vi "Module (Top Level).vi"(8 "error in":errorcluster) -> (0 "error out":errorcluster)   [LabVIEW 2017, in "Game.lvlib"]
uses:
  Game.lvlib
  User Events/TypeDefs/Shutdown UE FGV Command.ctl
  Global TypeDefs/Registered Modules.ctl
  Public TypeDefs/Messages.ctl
  Public TypeDefs/Module Events.ctl
  Libraries/TypeDefs/WorkspaceConfig.ctl
  Libraries/TypeDefs/UserInfo.ctl
  Libraries/TypeDefs/ServerStreamData.ctl
  Libraries/TypeDefs/HandPosition.ctl
  Libraries/TypeDefs/ElbowPosition.ctl
  Libraries/TypeDefs/ShoulderPosition.ctl
  Libraries/TypeDefs/UserInput.ctl
  Public TypeDefs/Target Position.ctl
  Logger/Logger.lvlib
  Error Handler/Error Handler.lvlib
  Controller/Controller.lvlib
  Libraries/GameComms.lvlib
  mypam/myPAM.lvlib
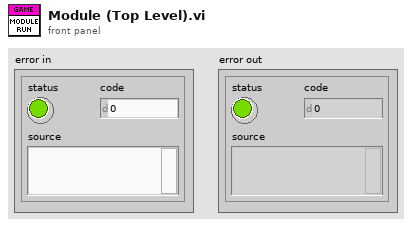
[diagram p1: front panel]
types:
  T1 = typedef "Registered Modules.ctl" = enum16{"Controller", "DAQ", "Error Handler", "Game", "myPAM", "WinHost", "Logger"}
  T2 = typedef "Shutdown UE FGV Command.ctl" = enum16{"create", "get", "destroy"}
  T3 = typedef "Controller.lvlib/Module Reference.ctl" = cluster{"calling module":T1, "module queues":T4, "module notifiers":T5}
  T4 = typedef "Controller.lvlib/Module Queues.ctl" = cluster{"message queue":refnum<queue>}
  T5 = typedef "Controller.lvlib/Module Notifiers.ctl" = cluster{"dummy notifier":refnum<notifier>}
  T6 = typedef "myPAM.lvlib/Module Reference.ctl" = cluster{"calling module":T1, "module queues":T7, "module notifiers":T8}
  T7 = typedef "myPAM.lvlib/Module Queues.ctl" = cluster{"message queue":refnum<queue>}
  T8 = typedef "myPAM.lvlib/Module Notifiers.ctl" = cluster{"end eff. pos.":refnum<notifier>}
  T9 = typedef "Logger.lvlib/Module Reference.ctl" = cluster{"calling module":T1, "module queues":T10, "module notifiers":T11}
  T10 = typedef "Logger.lvlib/Module Queues.ctl" = cluster{"message queue":refnum<queue>}
  T11 = typedef "Logger.lvlib/Module Notifiers.ctl" = cluster{"dummy notifier":refnum<notifier>}
  T12 = typedef "Game.lvlib/Module Reference.ctl" = cluster{"calling module":T1, "module queues":T13, "module notifiers":T14}
  T13 = typedef "Game.lvlib/Module Queues.ctl" = cluster{"message queue":refnum<queue>}
  T14 = typedef "Game.lvlib/Module Notifiers.ctl" = cluster{"dummy notifier":refnum<notifier>}
  T15 = typedef "Error Handler.lvlib/Module Reference.ctl" = cluster{"calling module":T1, "module queues":T16, "module notifiers":T17}
  T16 = typedef "Error Handler.lvlib/Module Queues.ctl" = cluster{"message queue":refnum<queue>}
  T17 = typedef "Error Handler.lvlib/Module Notifiers.ctl" = cluster{"dummy notifier":refnum<notifier>}
  T18 = typedef "Game.lvlib/Module Events.ctl" = enum16{"client connected", "client status change", "client disconnected"}
  T19 = typedef "Game.lvlib/GameComms.lvlib/ServerStreamData.ctl" = cluster{"hPos":T20, "ePos":T21, "sPos":T22, "uInput":T23}
  T20 = typedef "Game.lvlib/GameComms.lvlib/HandPosition.ctl" = cluster{"x":dbl, "y":dbl, "z":dbl}
  T21 = typedef "Game.lvlib/GameComms.lvlib/ElbowPosition.ctl" = cluster{"x":dbl, "y":dbl, "z":dbl}
  T22 = typedef "Game.lvlib/GameComms.lvlib/ShoulderPosition.ctl" = cluster{"x":dbl, "y":dbl, "z":dbl}
  T23 = typedef "Game.lvlib/GameComms.lvlib/UserInput.ctl" = cluster{"g":dbl}
  T24 = typedef "Game.lvlib/Target Position.ctl" = cluster{"x (mm)":dbl, "y (mm)":dbl}
  T25 = typedef "Game.lvlib/Messages.ctl" = enum16{"wait for client", "communicate", "shutdown"}
  T26 = typedef "Game.lvlib/GameComms.lvlib/UserInfo.ctl" = cluster{"id":string, "disabilityLevel ":dbl, "upperArmLength":dbl, "lowerArmLength":dbl}
  T27 = typedef "Game.lvlib/GameComms.lvlib/WorkspaceConfig.ctl" = cluster{"x":dbl, "y":dbl, "z":dbl}
  T28 = typedef "Game.lvlib/GameComms.lvlib/Connection.ctl" = cluster{"UDP Connection ID":refnum<k16>, "TCP Connection ID":refnum<k5>, "Remote UDP Port":u16, "Remote IP":u32}
  T29 = typedef "Game.lvlib/GameComms.lvlib/ClientStreamData.ctl" = cluster{"tPos":T30, "tWeight":dbl, "f":T31, "v":dbl}
  T30 = typedef "Game.lvlib/GameComms.lvlib/TargetPosition.ctl" = cluster{"x":dbl, "y":dbl, "z":dbl}
  T31 = typedef "Game.lvlib/GameComms.lvlib/ForceVector.ctl" = cluster{"x":dbl, "y":dbl, "z":dbl}
  T32 = typedef "Game.lvlib/GameComms.lvlib/ClientStatusData.ctl" = cluster{"gameState":u16, "playerName":string, "playerScore":dbl, "gameUnits":string}
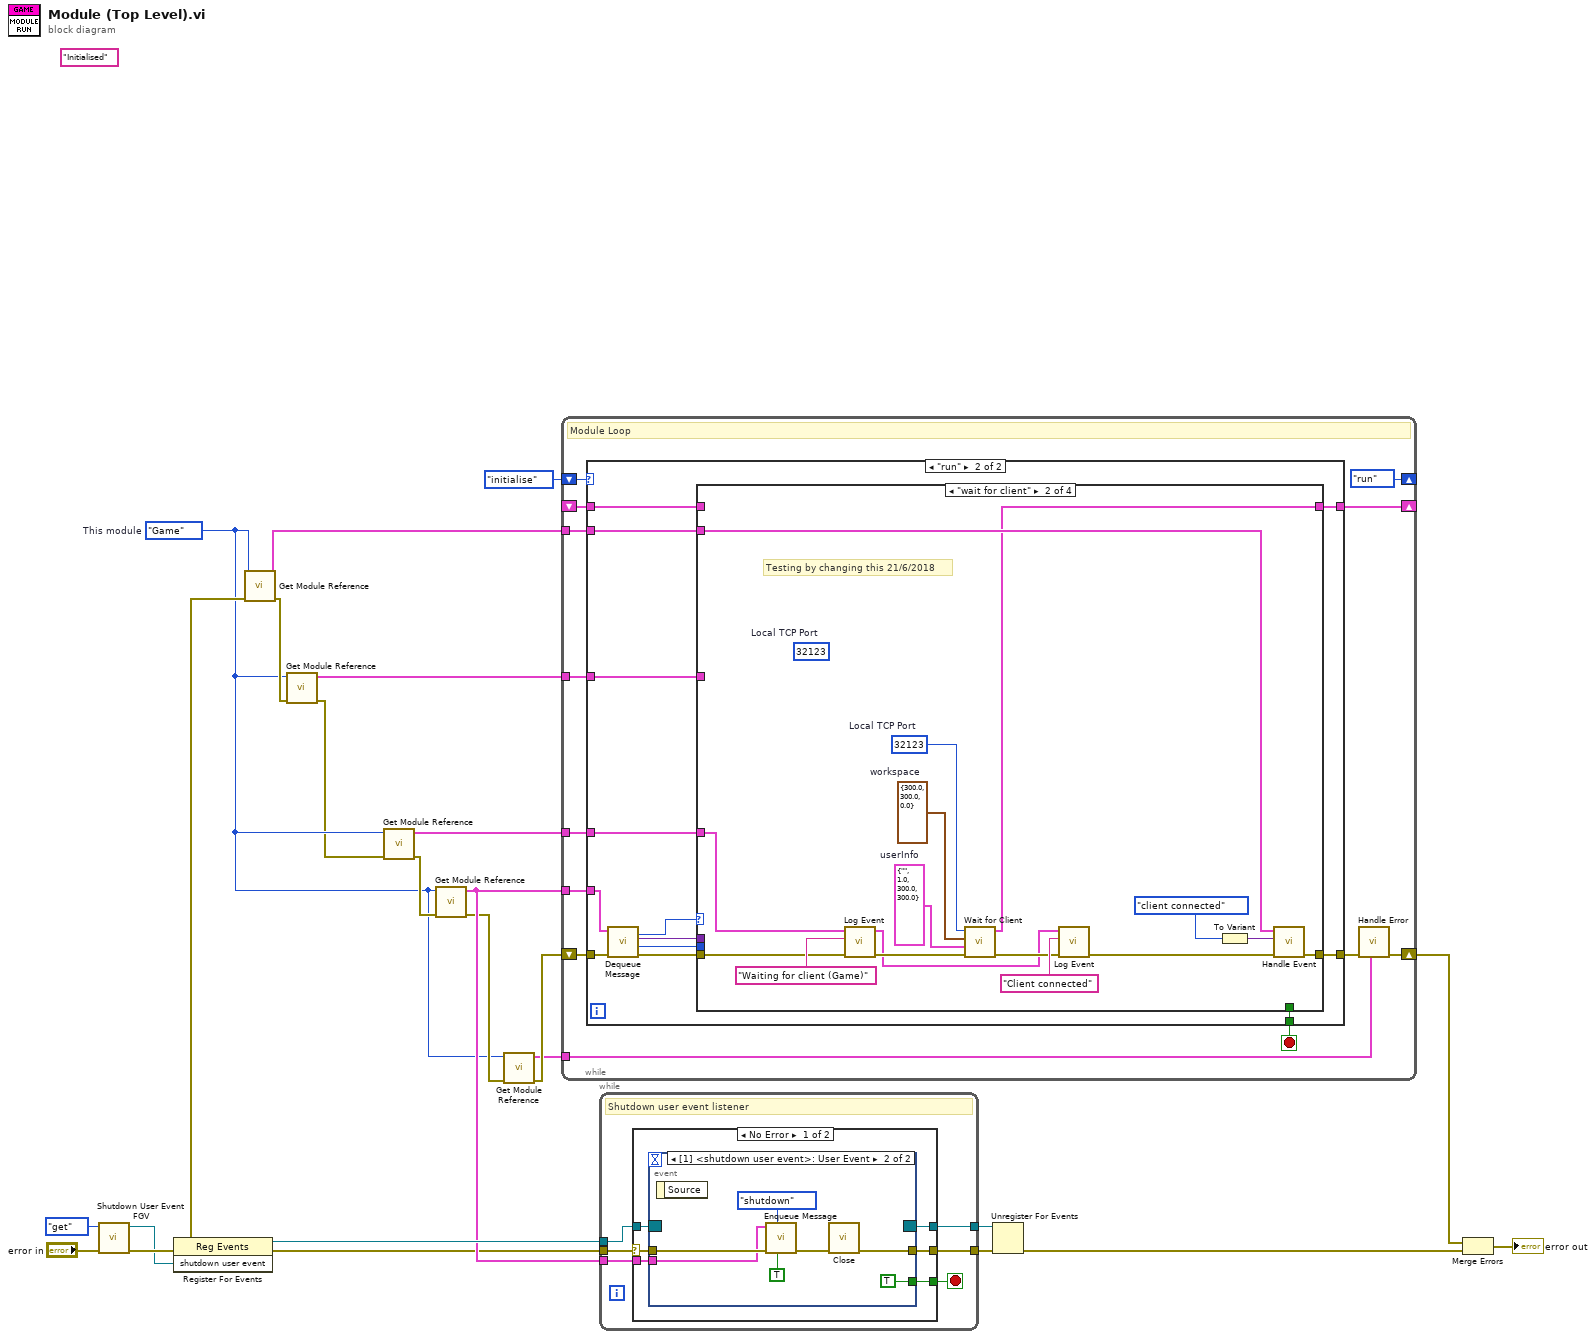
[diagram p0: block diagram]
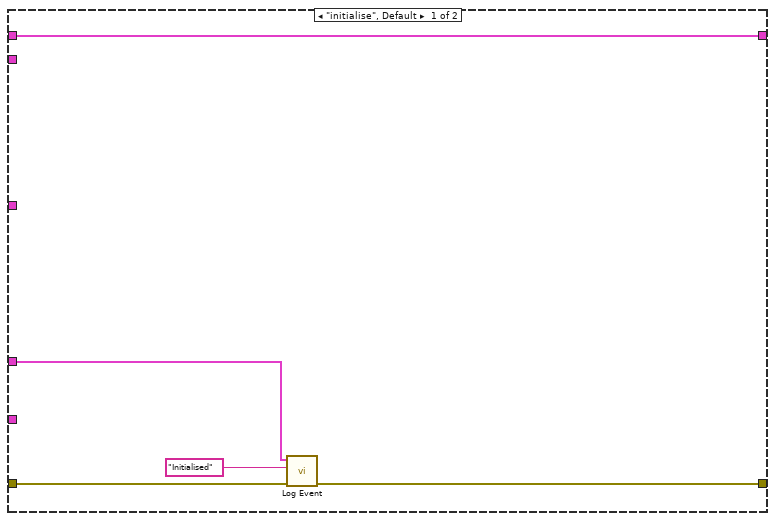
[diagram p2: hidden frame]
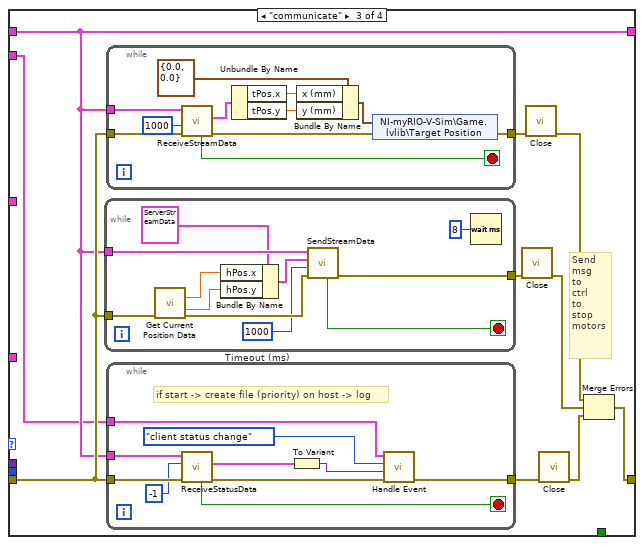
[diagram p4: hidden frame]
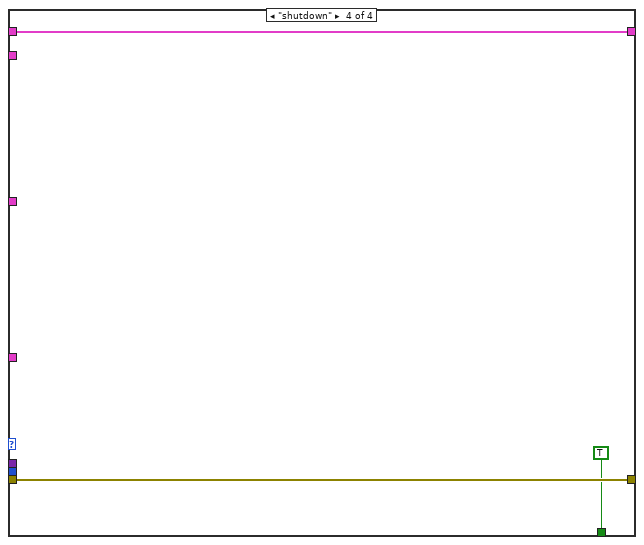
[diagram p5: hidden frame]
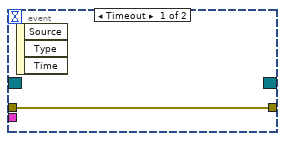
[diagram p6: hidden frame]
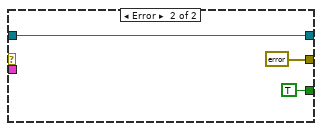
[diagram p7: hidden frame]
diagram:
  (unwired) "Initialised" ("string")
  w2 = Registered_Modules."Game"  # This module
  n1 = call "Shutdown User Event FGV.vi"("error in"="error in", "command"=Shutdown_UE_FGV_Command."get" ("Command")) -> ("error out"=w18:errorcluster, "shutdown user event"=w17:refnum<user-event>)  [unwired: 8 in]
  n2 = register-events(error in=w18, w17) -> (reference out=w22:refnum<event-registration>, error out=w6:errorcluster)  [unwired: 1 in]
  n3 = call "Get Module Reference.vi"("error in"=w6, "calling module"=w2) -> ("error out"=w4:errorcluster, "module reference"=w5:T3)  [unwired: 8 in]
  n4 = call "Get Module Reference.vi"("error in"=w4, "calling module"=w2) -> ("error out"=w1:errorcluster, "module reference"=w3:T6)  [unwired: 8 in]
  n5 = call "Get Module Reference.vi"("error in"=w1, "calling module"=w2) -> ("error out"=w8:errorcluster, "module reference"=w7:T9)  [unwired: 8 in]
  n6 = call "Get Module Reference.vi"("error in"=w8, "calling module"=w2) -> ("error out"=w11:errorcluster, "module reference"=w13:T12)  [unwired: 8 in]
  n7 = call "Get Module Reference.vi"("error in"=w11, "calling module"=w2) -> ("error out"=w10:errorcluster, "module reference"=w9:T15)  [unwired: 8 in]
  n8 = while {
    shift-right: [w33] -> w20
    shift-left: w10 -> [w30]
    tunnel: w13 -> [w36]
    shift-right: [enum16{"initialise", "run"}."run"] -> _
    shift-left: enum16{"initialise", "run"}."initialise" -> [w35]
    tunnel: w9 -> [w29]
    tunnel: w7 -> [w28]
    tunnel: w5 -> [w27]
    tunnel: w3 -> [w26]
    shift-right: [w25] -> _
    shift-left: _ -> [w24]
    stop <- w32 stop-if-true
    # "Module Loop"
    n9 = case shown="\"run\"" w35 {
      tunnel: [w38 w54] -> w34
      tunnel: w36 -> [_ w47]
      tunnel: [_ w49] -> w32
      tunnel: w30 -> [w41 w48]
      tunnel: w28 -> [w40 w46]
      tunnel: w27 -> [_ w45]
      tunnel: w26 -> [_ w44]
      tunnel: [w37 w43] -> w25
      tunnel: w24 -> [w37 w42]
      frame "initialise", Default {
        n10 = call "Log Event.vi"("error in"=w41, "event"="Initialised", "module reference in"=w40) -> ("error out"=w38:errorcluster)  [unwired: 7 in, 1 out]
      }
      frame "run" {
        n11 = call "Dequeue Message.vi"("error in"=w48, "module reference in"=w47) -> ("error out"=w52:errorcluster, "source"=w50:T1, "data"=w51:variant, "message"=w53:T25)  [unwired: 5 in, 1 out]
        n12 = case shown="\"wait for client\"" w53 {
          tunnel: [w56 w60 w76 w117] -> w54
          tunnel: w52 -> [w56 w68 w82 w117]
          tunnel: w51 -> [_ _ _ _]
          tunnel: w50 -> [_ _ _ _]
          tunnel: [_ _ _ TRUE] -> w49
          tunnel: w46 -> [_ w63 _ _]
          tunnel: w45 -> [_ w70 w74 _]
          tunnel: w44 -> [_ _ _ _]
          tunnel: [w55 w62 w75 w115] -> w43
          tunnel: w42 -> [w55 _ w75 w115]
          frame Default {
          }
          frame "wait for client" {
            (unwired) u16 32123  # Local TCP Port
            w64 = T26 {"id"="", "disabilityLevel "=1.0, "upperArmLength"=300.0, "lowerArmLength"=300.0}  # userInfo
            w65 = T27 {"x"=300.0, "y"=300.0, "z"=0.0}  # workspace
            w66 = u16 32123  # Local TCP Port
            # "Testing by changing this 21/6/2018"
            n13 = call "Log Event.vi"("error in"=w68, "event"="Waiting for client (Game)", "module reference in"=w63) -> ("error out"=w67:errorcluster, "module reference out"=w57:T9)  [unwired: 7 in]
            n14 = call "Wait for Client.vi"("Error In"=w67, "userInfo"=w64, "workspace"=w65, "Local TCP Port"=w66) -> ("Error Out"=w59:errorcluster, "Connection"=w62:T28)  [unwired: 6 in]
            n15 = call "Log Event.vi"("error in"=w59, "event"="Client connected", "module reference in"=w57) -> ("error out"=w58:errorcluster)  [unwired: 7 in, 1 out]
            n16 = To Variant(anything=Module_Events."client connected" ("module events")) -> (Variant=w71:variant)
            n17 = call "Handle Event.vi"("error in"=w58, "event"=w71, "module reference in"=w70) -> ("error out"=w60:errorcluster)  [unwired: 7 in, 1 out]
          }
          frame "communicate" {
            # "Send\nmsg\nto\nctrl\nto\nstop\nmotors"
            n18 = while {
              tunnel: w75 -> [w102]
              tunnel: w82 -> [w100]
              tunnel: [w101] -> w80
              stop <- w103 stop-if-true
              w98 = 1000  # Timeout (ms)
              n19 = call "Get Current Position Data.vi"("error in"=w100) -> ("link 2 x (mm)"=w96:dbl, "link 2 y (mm)"=w95:dbl, "error out"=w99:errorcluster)  [unwired: 10 in, 2 out]
              n20 = Bundle By Name(cluster=T19 {"hPos"={"x"=0.0, "y"=0.0, "z"=0.0}, "ePos"={"x"=0.0, "y"=0.0, "z"=0.0}, "sPos"={"x"=0.0, "y"=0.0, "z"=0.0}, "uInput"={"g"=0.0}} ("ServerStreamData"), "hPos.x"=w96, "hPos.y"=w95) -> (w94:T19)
              n21 = call "SendStreamData.vi"("Error In"=w99, "Timeout (ms)"=w98, "ServerStreamData"=w94, "Connection In"=w102) -> ("Error Out"=w101:errorcluster, "stop?"=w103:bool)  [unwired: 5 in, 1 out]
              n22 = Wait (ms)(milliseconds to wait=u32 8) -> ()  [unwired: 1 out]
            }
            n23 = while {
              tunnel: w75 -> [w113]
              tunnel: w82 -> [w112]
              tunnel: [w104] -> w81
              stop <- w114 stop-if-true
              n24 = call "ReceiveStreamData.vi"("Error In"=w112, "Timeout (ms)"=1000, "Connection In"=w113) -> ("Error Out"=w105:errorcluster, "ClientStreamData"=w110:T29, "stop?"=w114:bool)  [unwired: 5 in, 1 out]
              n25 = Unbundle By Name(w110) -> ("tPos.x"=w108:dbl, "tPos.y"=w107:dbl)
              n26 = Bundle By Name(cluster=T24 {"x (mm)"=0.0, "y (mm)"=0.0} ("Target Position"), "x (mm)"=w108, "y (mm)"=w107) -> (w106:T24)
              n27 = shared-variable "NI-myRIO-V-Sim\\Game.lvlib\\Target Position"(w106, error in=w105) -> (error out=w104:errorcluster)
            }
            n28 = while {
              tunnel: w75 -> [w91]
              tunnel: w82 -> [w90]
              tunnel: w74 -> [w88]
              tunnel: [w86] -> w73
              stop <- w92 stop-if-true
              # "if start -> create file (priority) on host -> log"
              n29 = call "ReceiveStatusData.vi"("error in"=w90, "Timeout (ms)"=-1, "Connection In"=w91) -> ("error out"=w87:errorcluster, "ClientStatusData"=w85:T32, "stop?"=w92:bool)  [unwired: 5 in, 1 out]
              n30 = To Variant(anything=w85) -> (Variant=w84:variant)
              n31 = call "Handle Event.vi"("error in"=w87, "data"=w84, "event"=Module_Events."client status change" ("module events"), "module reference in"=w88) -> ("error out"=w86:errorcluster)  [unwired: 6 in, 1 out]
            }
            n32 = call "Close.vi"("error in"=w80) -> ("error out"=w78:errorcluster)  [unwired: 10 in]
            n33 = call "Close.vi"("error in"=w81) -> ("error out"=w77:errorcluster)  [unwired: 10 in]
            n34 = call "Close.vi"("error in"=w73) -> ("error out"=w79:errorcluster)  [unwired: 10 in]
            n35 = Merge Errors(w77, w78, w79) -> (w76:errorcluster)
          }
          frame "shutdown" {
          }
        }
      }
    }
    n36 = call "Handle Error.vi"("module reference in"=w29, "error in"=w34) -> ("error out"=w33:errorcluster)  [unwired: 9 in]
  }
  n37 = while {
    tunnel: w22 -> [w123]
    tunnel: [w122] -> w21
    tunnel: w6 -> [w120]
    tunnel: [w119] -> w15
    tunnel: w13 -> [w118]
    stop <- w121 stop-if-true
    # "Shutdown user event listener"
    n38 = case shown="No Error" w120 {
      selector: w120 -> [w126 _]
      tunnel: w123 -> [w129 w139]
      tunnel: [w128 w139] -> w122
      tunnel: [w127 TRUE] -> w121
      tunnel: [w125 errorcluster {"status"=FALSE, "code"=0, "source"=""} ("error out")] -> w119
      tunnel: w118 -> [w124 _]
      frame No Error {
        n39 = event shown="[1] <shutdown user event>: User Event" {
          selector: w129 -> [_ _]
          dyn-events: [_ _] -> w128
          timeout: _ -> [_ _]
          tunnel: w126 -> [w130 w135]
          tunnel: [w130 w131] -> w125
          tunnel: [_ TRUE] -> w127
          tunnel: w124 -> [_ w134]
          event Timeout {
            n40 = event-data() -> ()  [unwired: 1 in, 3 out]
          }
          event User Event {
            n41 = event-data() -> ()  [unwired: 1 in, 1 out]
            n42 = call "Enqueue Message.vi"("high priority"=TRUE, "message"=Messages."shutdown", "error in"=w135, "module reference in"=w134) -> ("error out"=w132:errorcluster)  [unwired: 6 in, 1 out]
            n43 = call "Close.vi"("error in"=w132) -> ("error out"=w131:errorcluster)  [unwired: 10 in]
          }
        }
      }
      frame Error {
      }
    }
  }
  n44 = Unregister For Events(event registration refnum=w21, error in=w15) -> (error out=w16:errorcluster)
  n45 = Merge Errors(w20, w16) -> (→"error out":errorcluster)
